vi "ConstructLogger.vi"(7 "Logger Name (Logger)":string="Logger", 8 "error in (no error)":errorcluster, 9 "Name":string[](array[string]), 10 "Handle":refnum<class "LoggingHandle.lvclass">[](array[class]), 11 "Min Level":T1[](array[typedef])) -> (0 "error out":errorcluster, 3 "RQMHLogger out":refnum<class "RQMHLogger.lvclass">)   [LabVIEW 2024, in "Logger.lvlib"]
uses:
  Logger.lvlib
  LogHandle/Interface/LoggingHandle.lvclass
  RQMHLogger/RQMHLogger.lvclass
  HandleHolder/HandleHolder.lvclass
  Singleton/RQMHLogSingleton.lvlib
  Shared/Level.ctl
  Shared/LoggerShared.lvlib
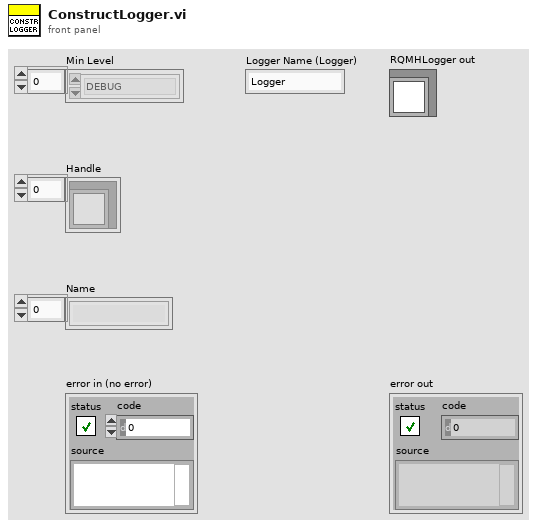
[diagram p1: front panel]
types:
  T1 = typedef "LoggerShared.lvlib/Level.ctl" = enum16{"DEBUG", "INFO", "WARNING", "ERROR", "CRITICAL"}
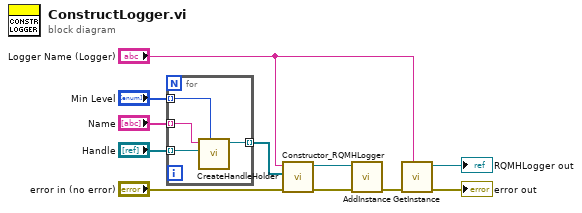
[diagram p0: block diagram]
diagram:
  n1 = for {
    tunnel: "Min Level" -> [w15] mode=indexing
    tunnel: "Handle" -> [w14] mode=indexing
    tunnel: "Name" -> [w13] mode=indexing
    tunnel: [w12] -> w8 mode=indexing
    n2 = call "CreateHandleHolder.vi"("Min Level"=w15, "Handle"=w14, "Name"=w13) -> ("HandleHolder out"=w12:refnum<class "HandleHolder.lvclass">)  [unwired: 8 in]
  }
  n3 = call "Constructor_RQMHLogger.vi"("error in (no error)"="error in (no error)", "Handles"=w8, "Name"="Logger Name (Logger)") -> ("error out"=w5:errorcluster, "RQMHLogger out"=w6:refnum<class "RQMHLogger.lvclass">)  [unwired: 7 in]
  n4 = call "AddInstance.vi"("error in (no error)"=w5, "RQMHLogger in"=w6) -> ("error out"=w4:errorcluster)  [unwired: 9 in]
  n5 = call "GetInstance.vi"("Logger Name (Logger)"="Logger Name (Logger)", "error in (no error)"=w4) -> ("error out"=→"error out":errorcluster, "RQMHLogger Get"=→"RQMHLogger out":refnum<class "RQMHLogger.lvclass">)  [unwired: 8 in]
